vi "Flatten Value.vi"(0 "Float In":refnum<class "Float.lvclass">, 11 "Error In":errorcluster) -> (4 "Float Out":refnum<class "Float.lvclass">, 8 "Value":string, 15 "Error Out":errorcluster)   [LabVIEW 2016, in "Float.lvclass"]
uses:
  Float.lvclass
  Float.lvclass/Float.ctl
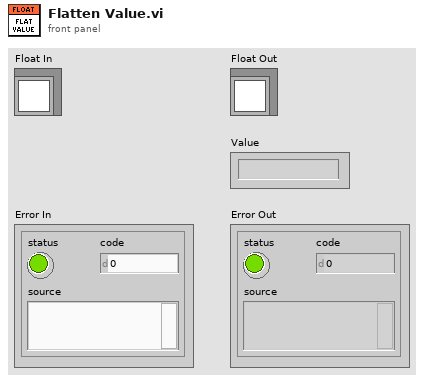
[diagram p1: front panel]
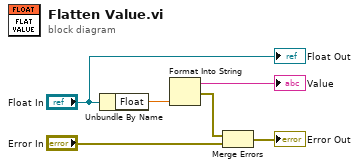
[diagram p0: block diagram]
diagram:
  n1 = Unbundle By Name("Float In") -> ("Float"=w5:dbl)
  n2 = Format Into String(w5) -> (resulting string=→"Value":string, error out=w3:errorcluster)  [unwired: 3 in]
  n3 = Merge Errors(w3, "Error In") -> (→"Error Out":errorcluster)
  "Float Out" <- "Float In"
